vi "HXG2_Re-Calc.vi"(8 "error in (no error)":errorcluster, 9 "Tube ID (in)":dbl, 10 "Target Re":dbl, 11 "Liq Tin (°F)":dbl) -> (0 "error out":errorcluster, 1 "Cp (BTU/lbm°F)":dbl, 2 "Density (lbm/ft³)":dbl, 3 "mdot (lbm/hr)":dbl, 4 "mu (lbm/ft*s)":dbl)   [LabVIEW 2012]
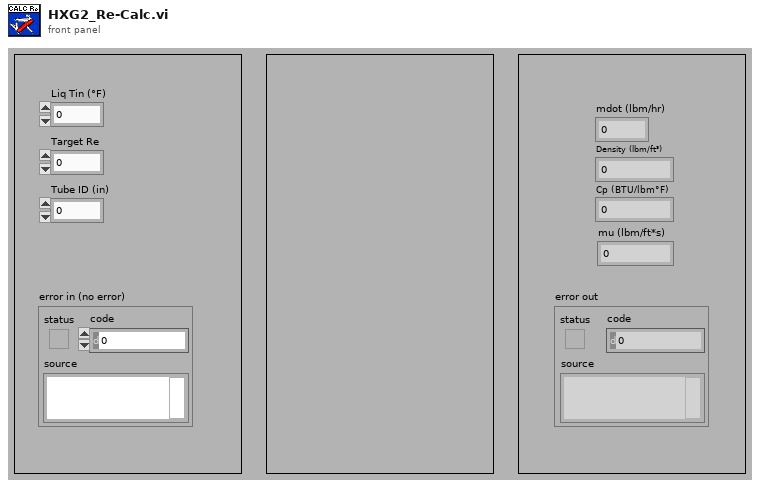
[diagram p1: front panel]
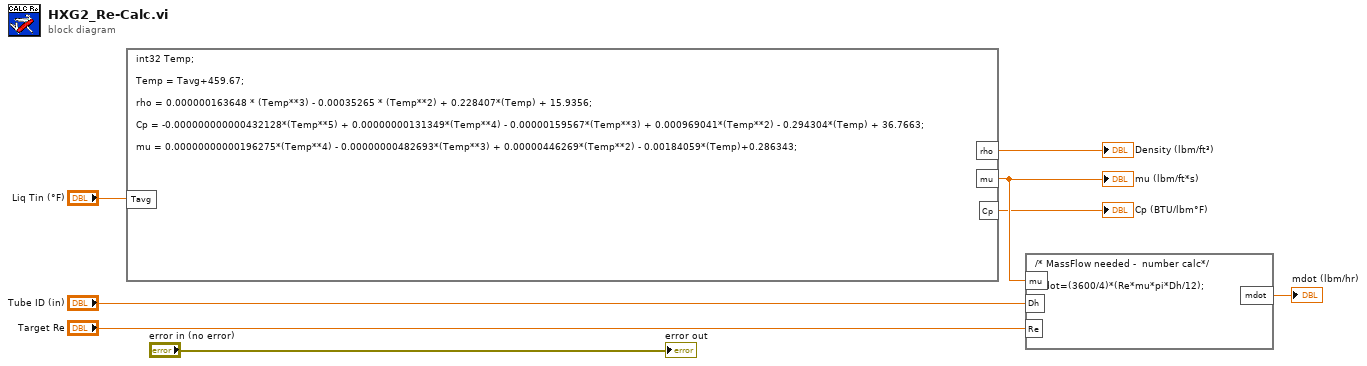
[diagram p0: block diagram]
diagram:
  n1 = formula code="int32 Temp;\n \nTemp = Tavg+459.67;\n\nrho = 0.000000163648 * (Temp**3) - 0.00035265 * (Temp**2) + 0.228407*(Temp) + 15.9356;\n\nCp = -0.000000000000432128*(Temp**5) + 0.00000000131349*(Temp**4) - 0.00000159567*(Temp**3) + 0.000969041*(Temp**2) - 0.294304*(Temp) + 36.7663;\n\nmu = 0.00000000000196275*(Temp**4) - 0.00000000482693*(Temp**3) + 0.00000446269*(Temp**2) - 0.00184059*(Temp)+0.286343;"("Tavg"="Liq Tin (°F)") -> ("rho"=→"Density (lbm/ft³)":dbl, "Cp"=→"Cp (BTU/lbm°F)":dbl, "mu"=w6:dbl)
  "mu (lbm/ft*s)" <- w6
  n2 = formula code="/* MassFlow needed -  number calc*/\n\nmdot=(3600/4)*(Re*mu*pi*Dh/12);"("Dh"="Tube ID (in)", "mu"=w6, "Re"="Target Re") -> ("mdot"=→"mdot (lbm/hr)":dbl)
  "error out" <- "error in (no error)"
